vi "test Filter.vi"() -> ()   [LabVIEW 2016]
uses:
  <vilib>/Analysis/1siggen.llb/Ramp Pattern by Delta.vi
  <vilib>/Analysis/3filter.llb/Equi-Ripple LowPass (DBL).vi
  <vilib>/Analysis/3filter.llb/Equi-Ripple HighPass (DBL).vi
  <vilib>/Analysis/NI_AALBase.lvlib
panel:
  out "High Pass":dbl[][](graph)
  out "Low Pass":dbl[][](graph)
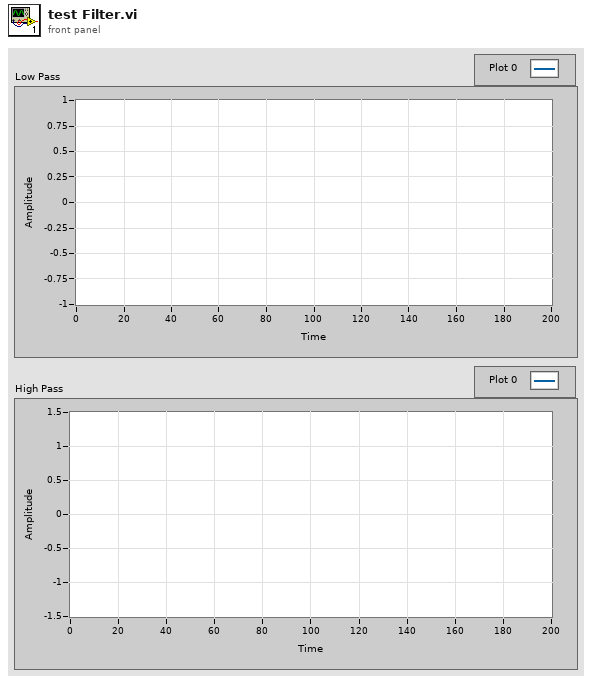
[diagram p1: front panel]
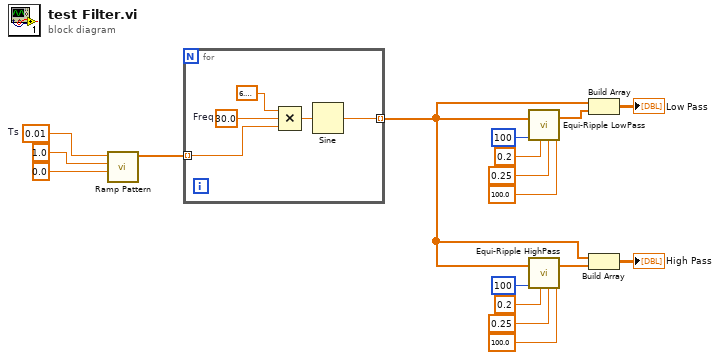
[diagram p0: block diagram]
diagram:
  w14 = 0.01  # Ts
  n1 = call-poly <vilib>:"Ramp Pattern.vi"("start"=0.0 ("end"), "end"=1.0, "delta"=w14) -> ("Ramp Pattern"=w13:dbl[])  [unwired: 6 in, 2 out]
  n2 = for {
    tunnel: w13 -> [w19] mode=indexing
    tunnel: [w18] -> w5 mode=indexing
    w20 = 30.0  # Freq
    n3 = Compound Arithmetic op=MULTIPLY(6.283185307179586, w20, w19) -> (w22:dbl)
    n4 = Sine(x=w22) -> (sin(x)=w18:dbl)
  }
  n5 = call-poly <vilib>:"Equi-Ripple LowPass.vi"("# of taps"=100, "pass freq"=0.2, "stop freq"=0.25, "sampling freq: fs"=100.0, "X"=w5) -> ("Filtered X"=w8:dbl[])  [unwired: 1 in, 1 out]
  n6 = call-poly <vilib>:"Equi-Ripple HighPass.vi"("# of taps"=100, "stop freq"=0.2, "high freq"=0.25, "sampling freq: fs"=100.0, "X"=w5) -> ("Filtered X"=w6:dbl[])  [unwired: 1 in, 1 out]
  n7 = Build Array(w5, w8) -> (→"Low Pass":dbl[][])
  n8 = Build Array(w5, w6) -> (→"High Pass":dbl[][])
